vi "get Wave Data.vi"(7 "data_size":u32, 8 "error in (no error)":errorcluster, 9 "values":u16, 10 "Board":u16, 11 "identifier":string) -> (0 "error out":errorcluster, 1 "values out":u16, 3 "function return":bool, 5 "data_size out":u32)   [LabVIEW 2015, in "XGL_DPP.lvlib"]
doc: "EXTERN DECLSPEC bool CALL_CONV getWaveData(const char * identifier,\n uint16_t Board,\n uint16_t * values,\n uint32_t * data_size\n);"
uses:
  XGL_DPP.lvlib
  XGL_DPP.dll
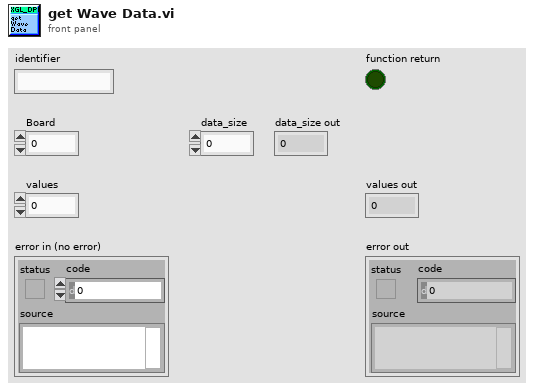
[diagram p1: front panel]
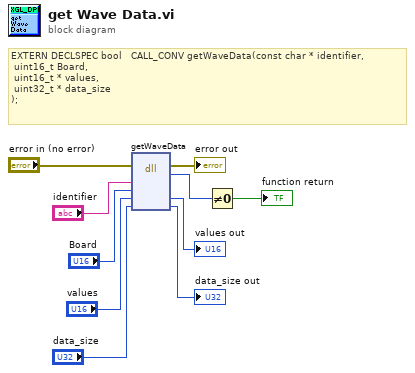
[diagram p0: block diagram]
diagram:
  # "EXTERN DECLSPEC bool   CALL_CONV getWaveData(const char * identifier,\n\tuint16_t Board,\n\tuint16_t * values,\n\tuint32_t * data_size\n);"
  n1 = dll-call lib="D:/Users/XRF/Desktop/Scanning Software_Demokritos_2015_v7/libs/Vis_2/XGL_DPP.*" fn="getWaveData"(error in="error in (no error)", "identifier"="identifier", "Board"="Board", "values"="values", "data_size"="data_size") -> (error out=→"error out":errorcluster, w9:u8, "values"=→"values out":u16, "data_size"=→"data_size out":u32)  [unwired: 4 in, 1 out]
  n2 = Not Equal To 0?(x=w9) -> (x != 0?=→"function return":bool)
